vi "PlotTestData.vi"(0 "TestDataTable Ref":refnum<vi>, 1 "StopPlotDataEvn":refnum<user-event>, 2 "CleanDataEvn":refnum<user-event>, 3 "Powers Ref":refnum<vi>[](array[refnum]), 5 "TestDataCurve Ref":refnum<vi>, 7 "XAxis Ref":refnum<vi>, 9 "YAxes Ref":refnum<vi>[](array[refnum]), 11 "TestData2D":refnum<vi>, 12 "Setting":T1={"TorqueSensor"={"Interface"="", "Read Unit"=enum."Kg.cm", "Encoder"=0, "Torque Filter"=0, "Max Torque"=2.0, "Max Power"=50.0, "Max Speed"=50.0, "Scale Factor CW"=2.0, "Scale Factor CCW"=2.0, "Scale Factor Zero"=2.0}, "TorqueSensorL"={"Interface"="", "Read Unit"=enum."Kg.cm", "Encoder"=0, "Torque Filter"=0, "Max Torque"=2.0, "Max Power"=50.0, "Max Speed"=50.0, "Scale Factor CW"=2.0, "Scale Factor CCW"=2.0, "Scale Factor Zero"=2.0}, "Power Meter"={"Wiring"=0, "Interface"="", "1P Mode"=1, "1P CurrentLimit"=0.0, "3P Mode"=1, "3P CurrentLimit"=0.0}, "Thermocouple"={"Interface"="", "value range"="T/C T type -100 ~ 400 degree C", "Channel Count"=8, "Limit 0"=0.0, "Limit 1"=0.0, "Limit 2"=0.0, "Limit 3"=0.0, "Limit 4"=0.0, "Limit 5"=0.0, "Limit 6"=0.0, "Limit 7"=0.0}, "DC-1000"={"Interface"=enum."AD-1"}, "ServoMotor"={"Interface"=enum."AD-1"}, "MotorDriver"={"D_Interface"="", "L_Interface"=""}, "TestMode"=enum."電子中軸測試", "PowerSupply"={"Interface"="", "Current"=50.0, "Voltage"=50.0}, "DUTMotor"={"Active"=FALSE, "TPCANBaudrate"=enum."PCAN_BAUD_1M 0x0014"}} {"Thermocouple"."Limit 7" format="%.1f"; "Thermocouple"."Limit 6" format="%.1f"; "Thermocouple"."Limit 5" format="%.1f"; "Thermocouple"."Limit 4" format="%.1f"; "Thermocouple"."Limit 3" format="%.1f"; "Thermocouple"."Limit 2" format="%.1f"; "Thermocouple"."Limit 1" format="%.1f"; "Thermocouple"."Limit 0" format="%.1f"; "Thermocouple"."Channel Count" min=0 max=24; "Power Meter"."3P Mode" items=["RMS", "MEAN", "DC"]; "Power Meter"."1P Mode" items=["RMS", "MEAN", "DC"]; "Power Meter"."Wiring" items=["1P2W", "1P2W+3P3W3M"]; "TorqueSensorL"."Scale Factor Zero" format="%#.6f"; "TorqueSensorL"."Scale Factor CCW" format="%#.6f"; "TorqueSensorL"."Scale Factor CW" format="%#.6f"; "TorqueSensorL"."Torque Filter" items=["OFF", "10Hz", "25Hz", "50Hz", "3Hz", "2Hz", "1Hz"]; "TorqueSensorL"."Encoder" items=["60-ppr"=60, "600-ppr"=600, "6000-ppr"=6000, "8192-ppr"=8192, "20-ppr"=20, "30-ppr"=30, "1-ppr"=1, "2-ppr"=2, "6-ppr"=6]; "TorqueSensor"."Scale Factor Zero" format="%#.6f"; "TorqueSensor"."Scale Factor CCW" format="%#.6f"; "TorqueSensor"."Scale Factor CW" format="%#.6f"; "TorqueSensor"."Torque Filter" items=["OFF", "10Hz", "25Hz", "50Hz", "3Hz", "2Hz", "1Hz"]; "TorqueSensor"."Encoder" items=["60-ppr"=60, "600-ppr"=600, "6000-ppr"=6000, "8192-ppr"=8192, "20-ppr"=20, "30-ppr"=30, "1-ppr"=1, "2-ppr"=2, "6-ppr"=6]}, 13 "DataVisible Ref":refnum<vi>, 14 "Efficiency Ref":refnum<vi>) -> ()   [LabVIEW 2024]
uses:
  MFActor/SystemSettings.ctl
  ref/PCAN/CAN Communication.llb/TPCANBaudrate.ctl
  PlotTestDataStep.ctl
  <vilib>/Utility/error.llb/Trim Whitespace One-Sided.vi
  Global Variables.vi
panel:
  out "TestData1D 2":dbl[](array[numeric])
  out "DataNumber":u32
  out "StartTime":u32
  out "TestDataCurve":dbl[][](array[numeric])
  out "TestData1D":dbl[](array[numeric])
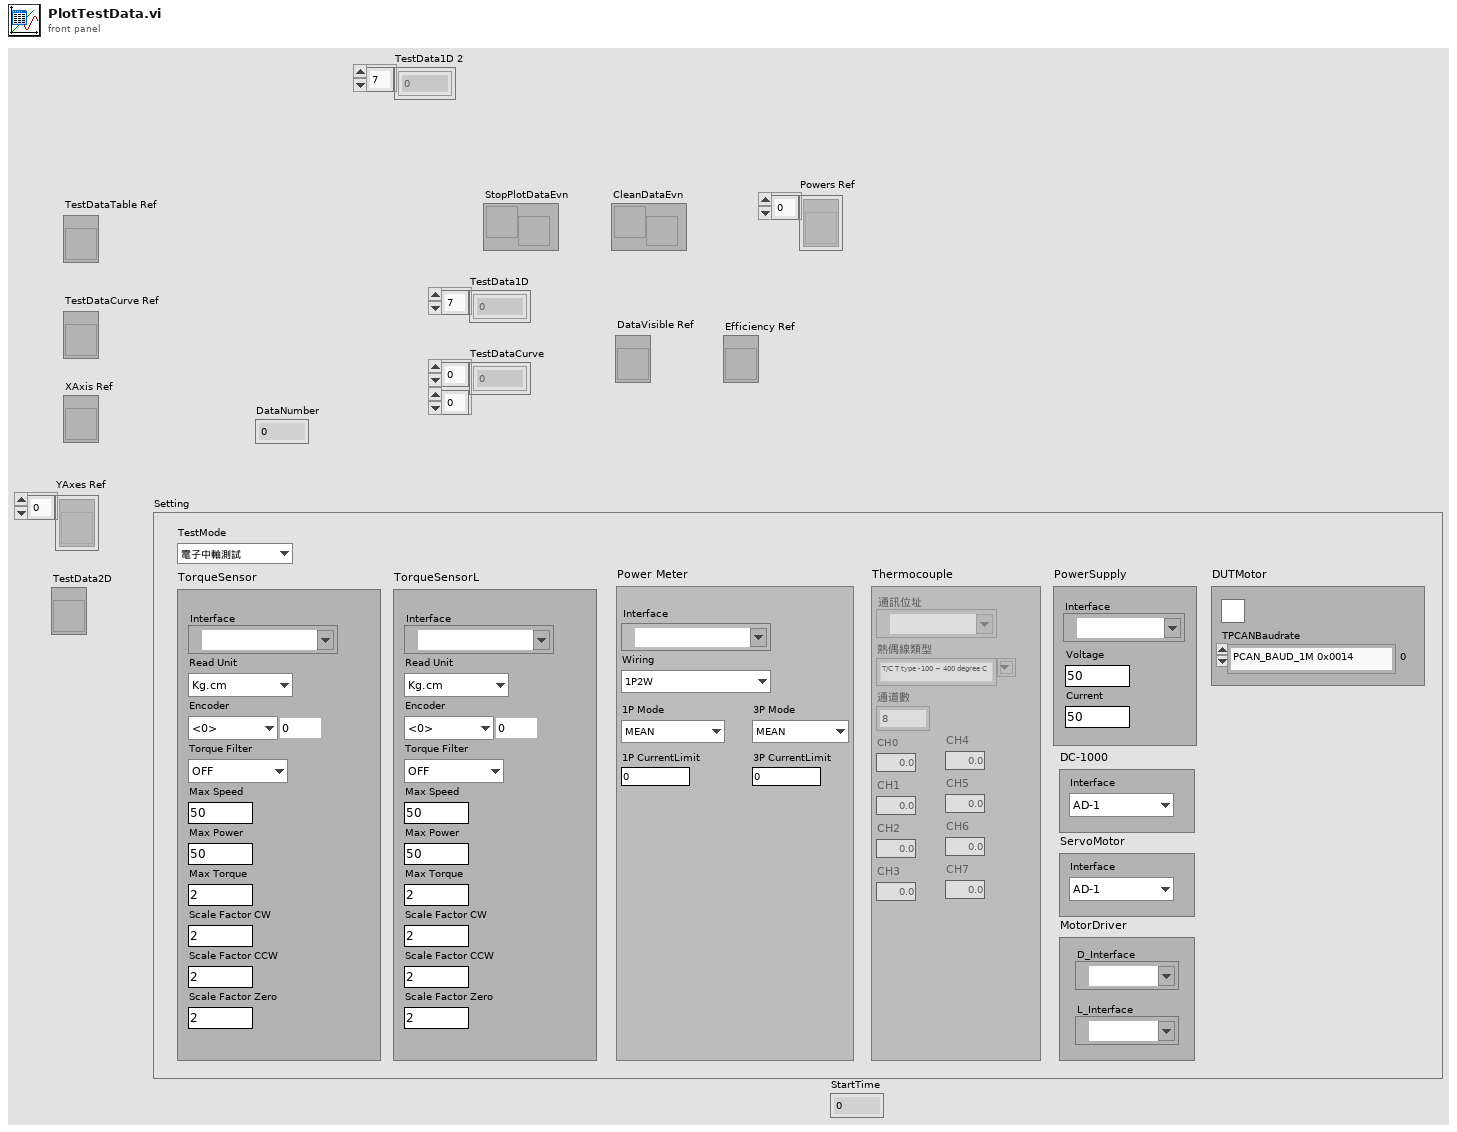
[diagram p1: front panel]
types:
  T1 = typedef "SystemSettings.ctl" = cluster{"TorqueSensor":cluster{"Interface":refnum<visa-resource-name>, "Read Unit":enum16{"oz.in", "oz.ft", "lb.in", "lb.ft", "g.cm", "Kg.cm", "mN.m", "cN.m", "N.m"}, "Encoder":u16, "Torque Filter":u16, "Max Torque":dbl, "Max Power":dbl, "Max Speed":dbl, "Scale Factor CW":dbl, "Scale Factor CCW":dbl, "Scale Factor Zero":dbl}, "TorqueSensorL":cluster{"Interface":refnum<visa-resource-name>, "Read Unit":enum16{"oz.in", "oz.ft", "lb.in", "lb.ft", "g.cm", "Kg.cm", "mN.m", "cN.m", "N.m"}, "Encoder":u16, "Torque Filter":u16, "Max Torque":dbl, "Max Power":dbl, "Max Speed":dbl, "Scale Factor CW":dbl, "Scale Factor CCW":dbl, "Scale Factor Zero":dbl}, "Power Meter":cluster{"Wiring":u16, "Interface":refnum<visa-resource-name>, "1P Mode":u16, "1P CurrentLimit":dbl, "3P Mode":u16, "3P CurrentLimit":dbl}, "Thermocouple":cluster{"Interface":refnum<visa-resource-name>, "value range":string, "Channel Count":i32, "Limit 0":dbl, "Limit 1":dbl, "Limit 2":dbl, "Limit 3":dbl, "Limit 4":dbl, "Limit 5":dbl, "Limit 6":dbl, "Limit 7":dbl}, "DC-1000":cluster{"Interface":enum16{"AD-0", "AD-1"}}, "ServoMotor":cluster{"Interface":enum16{"AD-0", "AD-1"}}, "MotorDriver":cluster{"D_Interface":refnum<visa-resource-name>, "L_Interface":refnum<visa-resource-name>}, "TestMode":enum16{"電子中軸測試", "中置電機測試"}, "PowerSupply":cluster{"Interface":refnum<visa-resource-name>, "Current":dbl, "Voltage":dbl}, "DUTMotor":cluster{"Active":bool, "TPCANBaudrate":T2}}
  T2 = typedef "TPCANBaudrate.ctl" = enum16{"PCAN_BAUD_1M 0x0014", "PCAN_BAUD_800K 0x0016", "PCAN_BAUD_500K 0x001C", "PCAN_BAUD_250K 0x011C", "PCAN_BAUD_125K 0x031C", "PCAN_BAUD_100K 0x432F", "PCAN_BAUD_95K 0xC34E", "PCAN_BAUD_83K 0x852B", "PCAN_BAUD_50K 0x472F", "PCAN_BAUD_47K 0x1414", "PCAN_BAUD_33K 0x8B2F", "PCAN_BAUD_20K 0x532F", "PCAN_BAUD_10K 0x672F", "PCAN_BAUD_5K 0x7F7F", "User Baudrate"}
  T3 = cluster{"GraphTestData":dbl[], "GraphTestData 2":dbl[]}[]
  T4 = typedef "PlotTestDataStep.ctl" = enum16{"None", "CheckTestData", "CalculateEffi", "Plot", "DataVisible", "UpdateGraph", "Clean", "End"}
  T5 = cluster{"SR":dbl, "EffiDriver":dbl, "EffiMotor":dbl, "EffiTotal":dbl}
  T6 = cluster{"TestDataCurve":dbl[], "TestDataCurve":dbl[]}
  T7 = cluster{"TestDataCurve":dbl[], "TestDataCurve":dbl[]}[]
  T8 = typedef "LVRowAndColumnUnsignedTypeDef.ctl" = cluster{"Row":u32, "Column":u32}
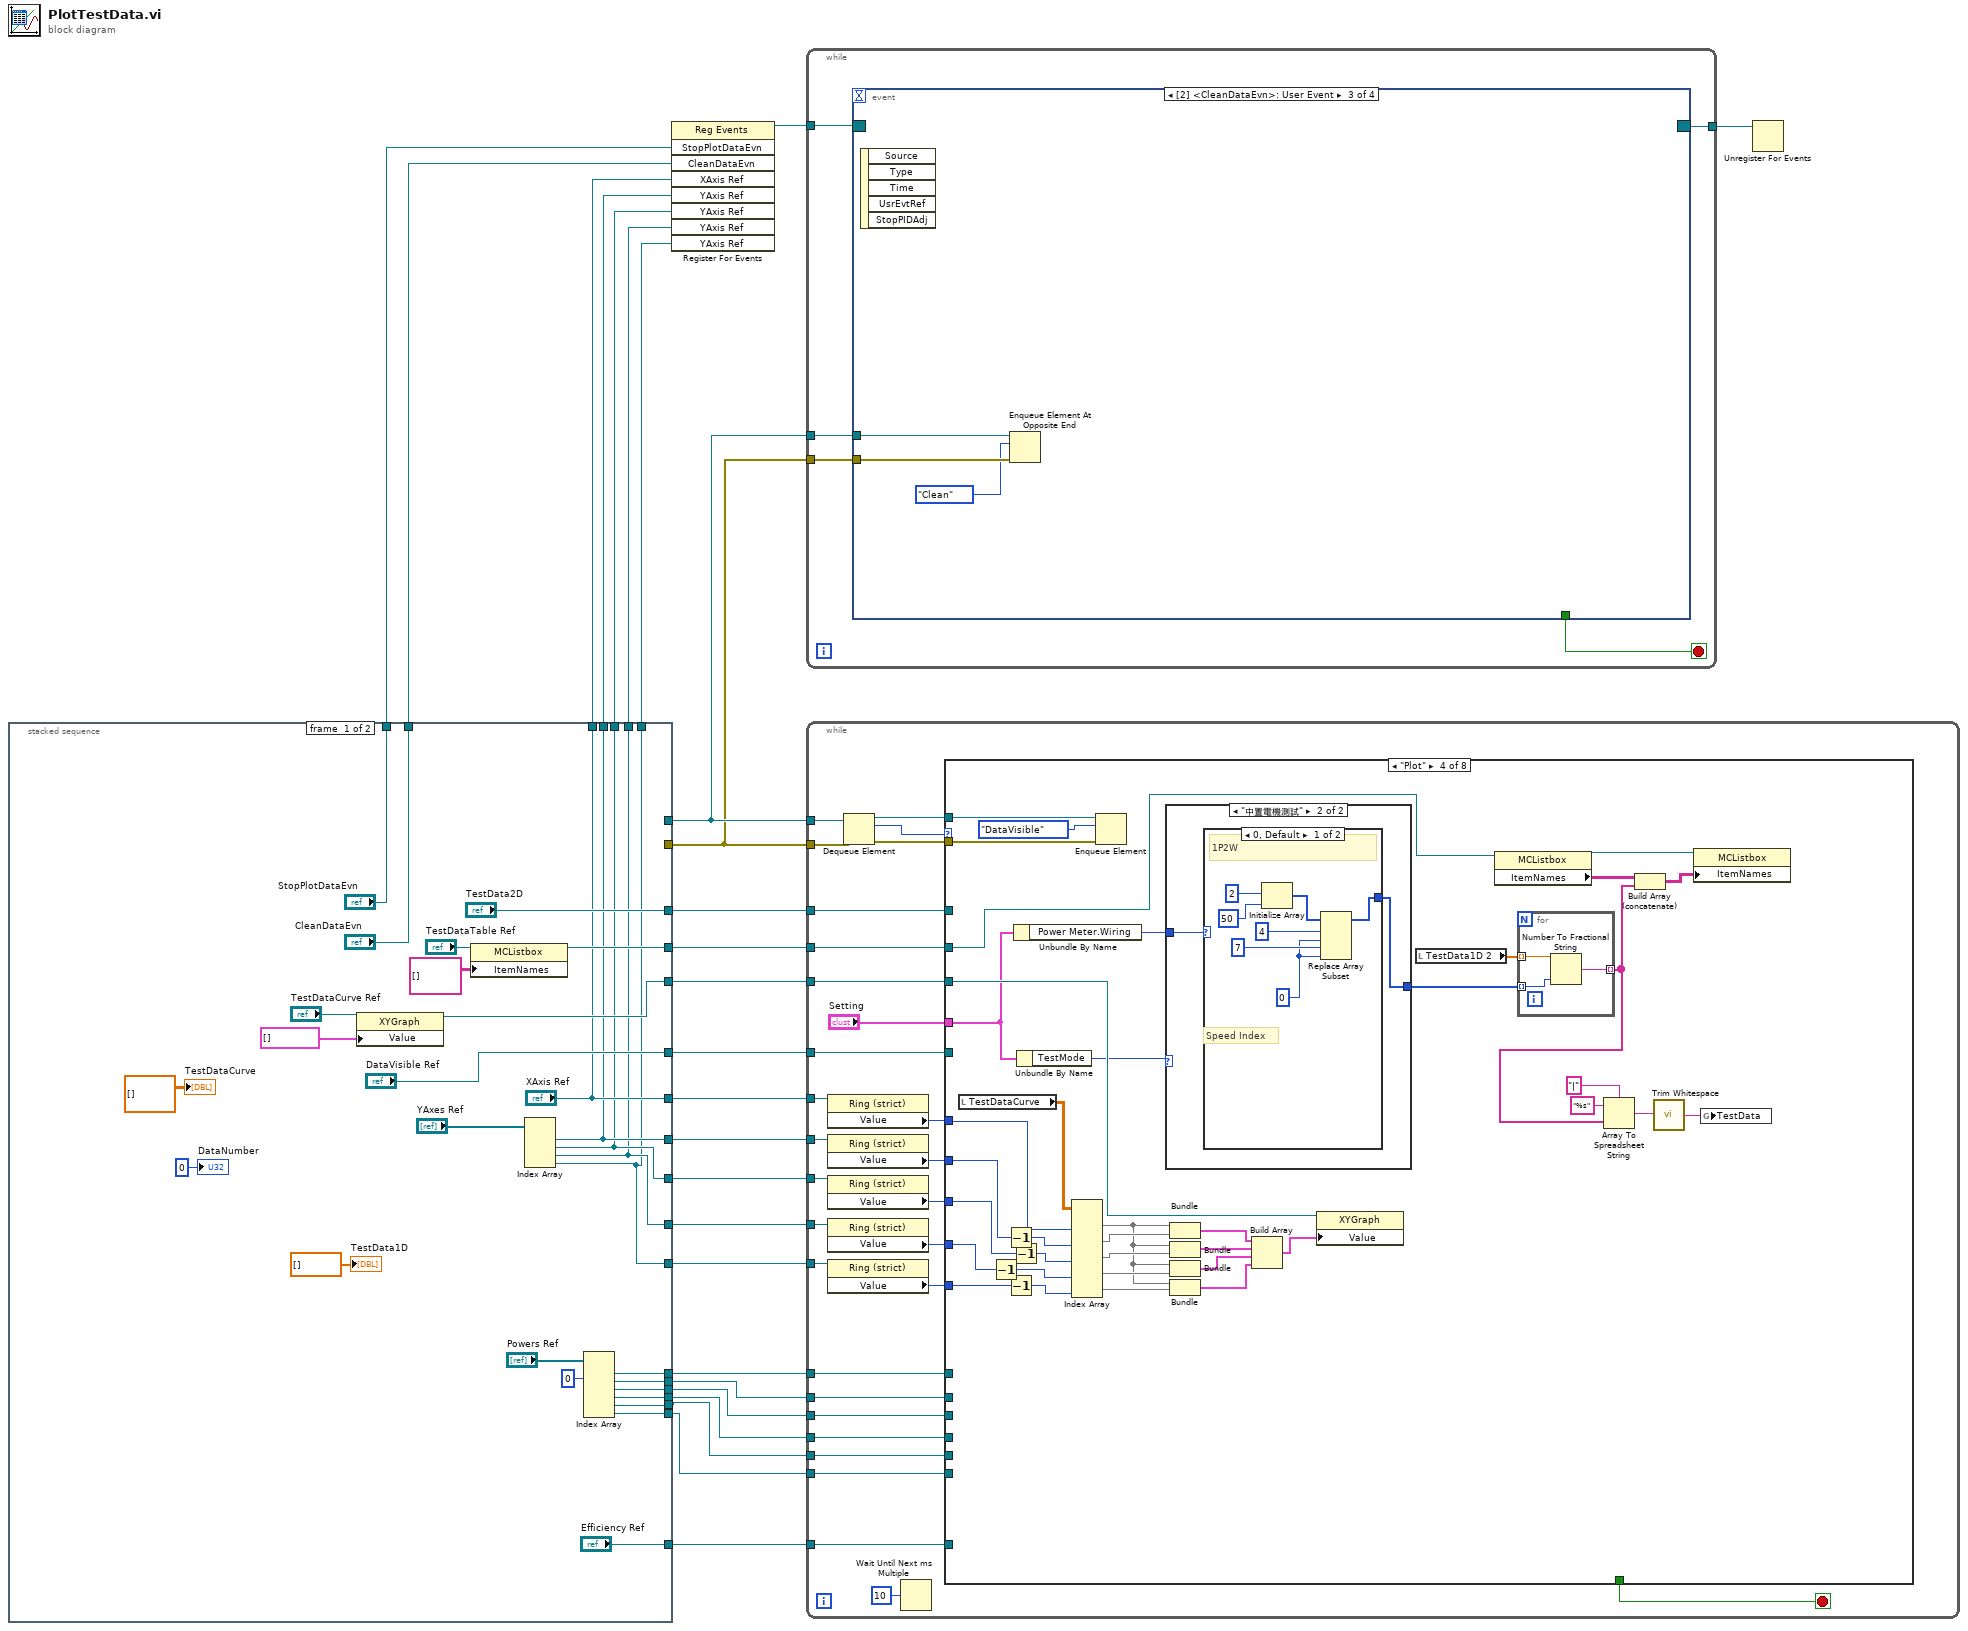
[diagram p0: block diagram]
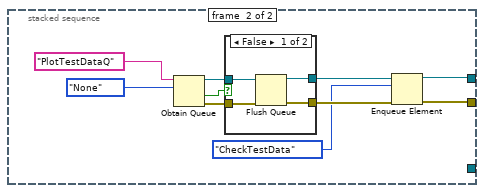
[diagram p2: hidden frame]
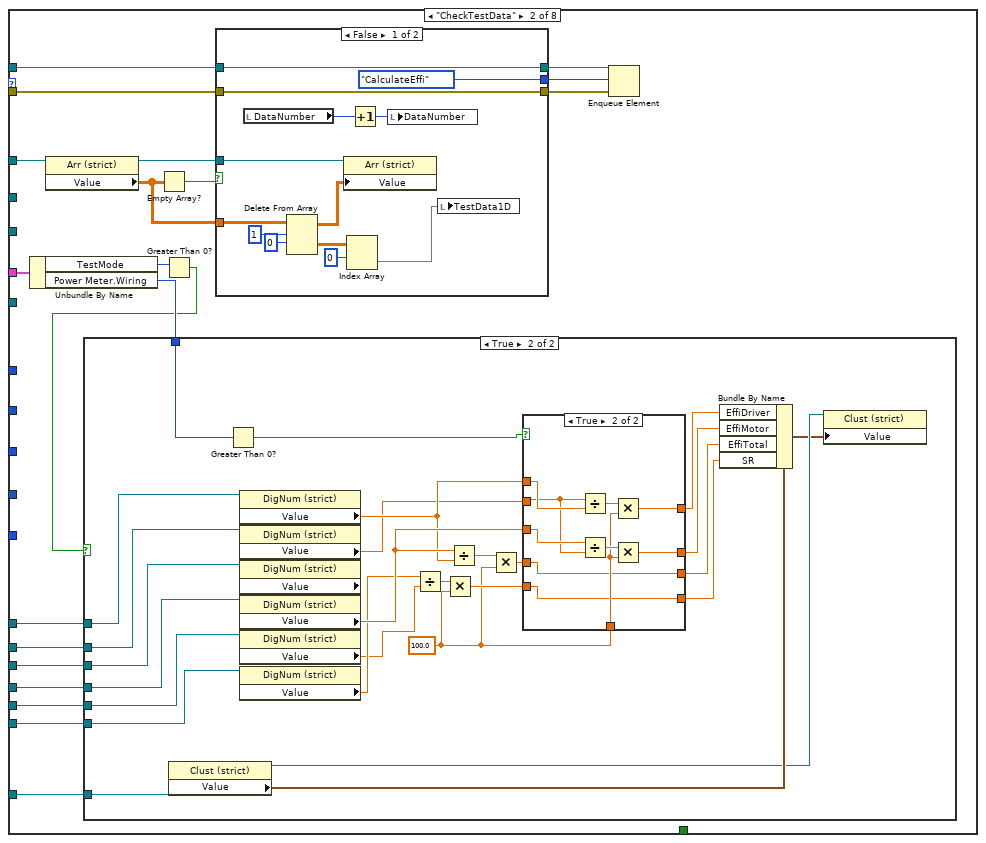
[diagram p5: hidden frame]
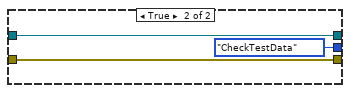
[diagram p8: hidden frame]
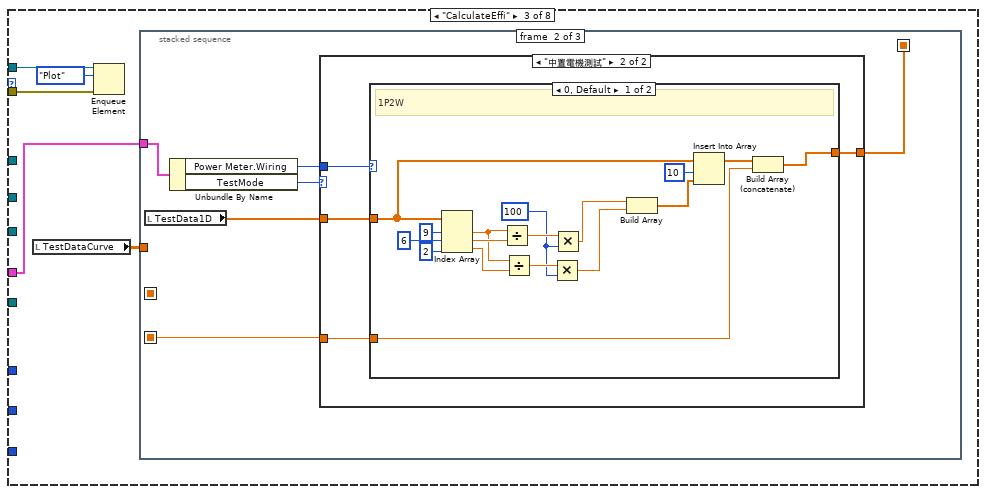
[diagram p9: hidden frame]
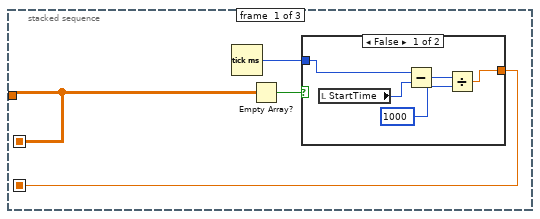
[diagram p10: hidden frame]
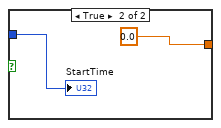
[diagram p11: hidden frame]
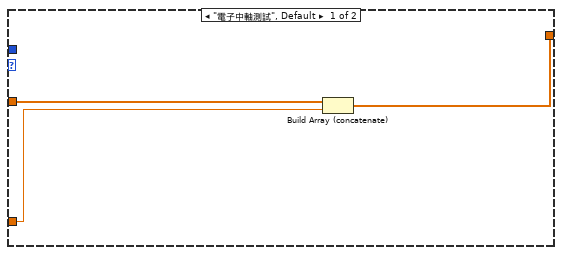
[diagram p12: hidden frame]
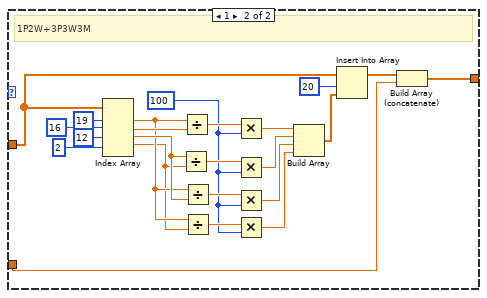
[diagram p13: hidden frame]
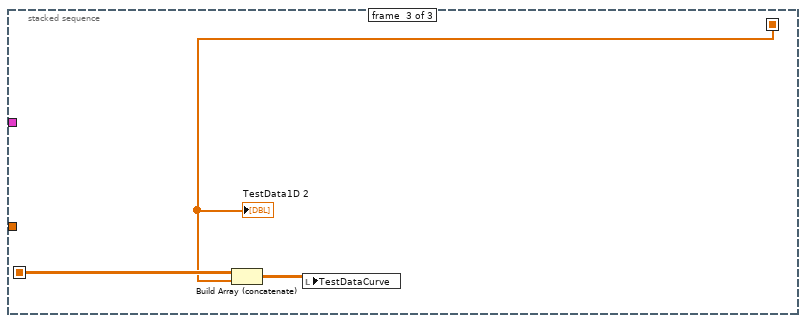
[diagram p14: hidden frame]
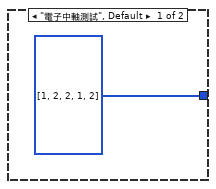
[diagram p15: hidden frame]
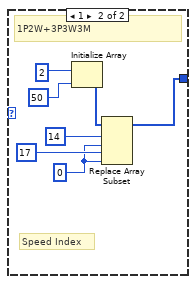
[diagram p16: hidden frame]
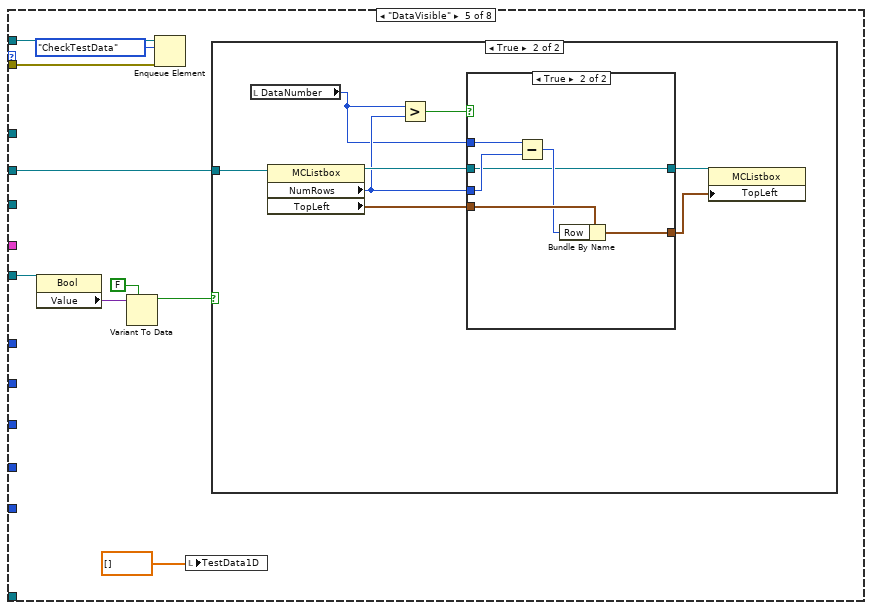
[diagram p17: hidden frame]
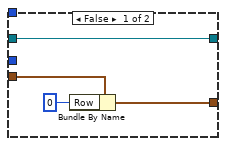
[diagram p19: hidden frame]
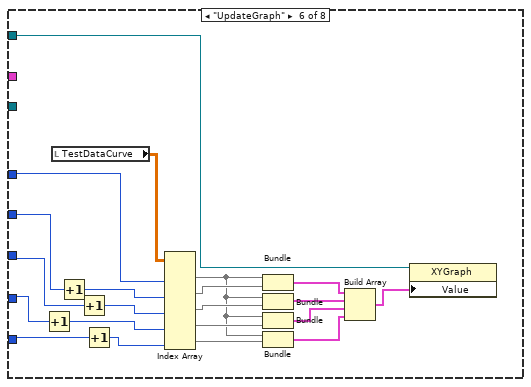
[diagram p20: hidden frame]
diagram:
  n1 = stacked-sequence {
    tunnel: ["StopPlotDataEvn" _] -> w27
    tunnel: ["CleanDataEvn" _] -> w26
    tunnel: [_ w58] -> w24
    tunnel: [_ w57] -> w23
    tunnel: ["TestData2D" _] -> w22
    tunnel: [w50 _] -> w21
    tunnel: [w47 _] -> w20
    tunnel: ["XAxis Ref" _] -> w19
    tunnel: [w41 _] -> w18
    tunnel: [w40 _] -> w17
    tunnel: [w39 _] -> w16
    tunnel: [w38 _] -> w15
    tunnel: ["DataVisible Ref" _] -> w13
    tunnel: ["XAxis Ref" _] -> w12
    tunnel: [w41 _] -> w11
    tunnel: [w40 _] -> w10
    tunnel: [w39 _] -> w9
    tunnel: [w38 _] -> w8
    tunnel: [w35 _] -> w7
    tunnel: [w34 _] -> w6
    tunnel: [w33 _] -> w5
    tunnel: [w32 _] -> w4
    tunnel: ["Efficiency Ref" _] -> w3
    tunnel: [w29 _] -> w2
    tunnel: [w28 _] -> w1
    frame #0 {
      n2 = property class="XYGraph"(reference="TestDataCurve Ref", "Value"=T3 []) -> (reference out=w47:refnum<vi>)  [unwired: 1 in, 1 out]
      n3 = property class="MCListbox"(reference="TestDataTable Ref", "ItemNames"=string[][] [] ("Item Names")) -> (reference out=w50:refnum<vi>)  [unwired: 1 in, 1 out]
      n4 = Index Array(array="YAxes Ref") -> (element #1=w41:refnum<vi>, element #2=w40:refnum<vi>, element #3=w39:refnum<vi>, element #4=w38:refnum<vi>)  [unwired: 4 in]
      n5 = Index Array(array="Powers Ref", index #1=0 ("index")) -> (element #1=w35:refnum<vi>, element #2=w34:refnum<vi>, element #3=w33:refnum<vi>, element #4=w32:refnum<vi>, element #5=w29:refnum<vi>, element #6=w28:refnum<vi>)  [unwired: 5 in]
      "TestDataCurve" <- dbl[][] [] ("TestData2D")
      "DataNumber" <- u32 0 ("DataNumber")
      "TestData1D" <- dbl[] [] ("TestData1D")
    }
    frame #1 {
      n6 = Obtain Queue(name (unnamed)="PlotTestDataQ", element data type=PlotTestDataStep."None" ("PlotTestDataStep")) -> (queue out=w62:refnum<queue>, created new?=w63:bool, error out=w61:errorcluster)  [unwired: 3 in]
      n7 = case shown="False" w63 {
        tunnel: w62 -> [w69 w71]
        tunnel: w61 -> [w68 w70]
        tunnel: [w67 w71] -> w60
        tunnel: [w66 w70] -> w59
        frame False {
          n8 = Flush Queue(queue=w69, error in (no error)=w68) -> (queue out=w67:refnum<queue>, error out=w66:errorcluster)  [unwired: 1 out]
        }
        frame True {
        }
      }
      n9 = Enqueue Element(queue=w60, element=PlotTestDataStep."CheckTestData", error in (no error)=w59) -> (queue out=w58:refnum<queue>, error out=w57:errorcluster)  [unwired: 1 in, 1 out]
    }
  }
  n10 = register-events(w27, w26, w12, w11, w10, w9, w8) -> (reference out=w25:refnum<event-registration>)  [unwired: 2 in, 1 out]
  n11 = while {
    tunnel: w25 -> [w76]
    tunnel: w24 -> [w75]
    tunnel: w23 -> [w74]
    tunnel: [w72] -> w14
    stop <- w73 stop-if-true
    n12 = event shown="[2] <CleanDataEvn>: User Event" {
      selector: w76 -> [_ _ _ _]
      dyn-events: [_ _ _ _] -> w72
      timeout: _ -> [_ _ _ _]
      tunnel: w75 -> [_ w82 w85 w88]
      tunnel: w74 -> [_ w81 w84 w87]
      tunnel: [_ TRUE _ _] -> w73
      event Timeout {
        n13 = event-data() -> ()  [unwired: 1 in, 3 out]
      }
      event User Event {
        n14 = event-data() -> ()  [unwired: 1 in, 5 out]
        n15 = Flush Queue(queue=w82, error in (no error)=w81) -> (queue out=w80:refnum<queue>, error out=w79:errorcluster)  [unwired: 1 out]
        n16 = Enqueue Element At Opposite End(queue=w80, element=PlotTestDataStep."End", error in (no error)=w79) -> ()  [unwired: 1 in, 3 out]
      }
      event User Event {
        n17 = event-data() -> ()  [unwired: 1 in, 5 out]
        n18 = Enqueue Element At Opposite End(queue=w85, element=PlotTestDataStep."Clean", error in (no error)=w84) -> ()  [unwired: 1 in, 3 out]
      }
      event Value Change {
        n19 = event-data() -> ()  [unwired: 1 in, 6 out]
        n20 = Enqueue Element(queue=w88, element=PlotTestDataStep."UpdateGraph", error in (no error)=w87) -> ()  [unwired: 1 in, 3 out]
      }
    }
  }
  n21 = while {
    tunnel: w24 -> [w117]
    tunnel: w23 -> [w116]
    tunnel: w22 -> [w110]
    tunnel: w21 -> [w108]
    tunnel: w20 -> [w97]
    tunnel: w19 -> [w99]
    tunnel: w18 -> [w107]
    tunnel: w17 -> [w106]
    tunnel: w16 -> [w105]
    tunnel: w15 -> [w104]
    tunnel: w13 -> [w96]
    tunnel: w7 -> [w94]
    tunnel: w6 -> [w93]
    tunnel: w5 -> [w92]
    tunnel: w4 -> [w91]
    tunnel: w3 -> [w95]
    tunnel: w2 -> [w90]
    tunnel: w1 -> [w89]
    stop <- w111 stop-if-true
    n22 = property class="Ring (strict)"(reference=w99) -> ("Value"=w98:u16)  [unwired: 1 in, 2 out]
    n23 = property class="Ring (strict)"(reference=w107) -> ("Value"=w103:u16)  [unwired: 1 in, 2 out]
    n24 = property class="Ring (strict)"(reference=w106) -> ("Value"=w102:u16)  [unwired: 1 in, 2 out]
    n25 = property class="Ring (strict)"(reference=w105) -> ("Value"=w101:u16)  [unwired: 1 in, 2 out]
    n26 = property class="Ring (strict)"(reference=w104) -> ("Value"=w100:u16)  [unwired: 1 in, 2 out]
    n27 = Dequeue Element(queue=w117, error in (no error)=w116) -> (queue out=w115:refnum<queue>, element=w113:T4, error out=w114:errorcluster)  [unwired: 1 in, 1 out]
    n28 = Wait Until Next ms Multiple(millisecond multiple=u32 10) -> ()  [unwired: 1 out]
    n29 = case shown="\"Plot\"" w113 {
      tunnel: w115 -> [_ w133 w196 w279 w325 _ _ w383]
      tunnel: w114 -> [_ w132 w195 w278 w324 _ _ w382]
      tunnel: [_ _ _ _ _ _ _ TRUE] -> w111
      tunnel: w110 -> [_ w137 _ _ _ _ _ _]
      tunnel: "Setting" -> [_ w124 w193 w276 _ _ _ _]
      tunnel: w108 -> [_ _ _ w299 w326 _ w376 _]
      tunnel: w103 -> [_ _ _ w294 _ w356 _ _]
      tunnel: w102 -> [_ _ _ w293 _ w357 _ _]
      tunnel: w101 -> [_ _ _ w292 _ w358 _ _]
      tunnel: w100 -> [_ _ _ w291 _ w359 _ _]
      tunnel: w98 -> [_ _ _ w265 _ w353 _ _]
      tunnel: w97 -> [_ _ _ w281 _ w354 w374 _]
      tunnel: w96 -> [_ _ _ _ w330 _ _ _]
      tunnel: w95 -> [_ w121 _ _ _ _ _ _]
      tunnel: w94 -> [_ w128 _ _ _ _ _ _]
      tunnel: w93 -> [_ w127 _ _ _ _ _ _]
      tunnel: w92 -> [_ w126 _ _ _ _ _ _]
      tunnel: w91 -> [_ w125 _ _ _ _ _ _]
      tunnel: w90 -> [_ w119 _ _ _ _ _ _]
      tunnel: w89 -> [_ w118 _ _ _ _ _ _]
      frame "None", Default {
      }
      frame "CheckTestData" {
        n30 = Unbundle By Name(w124) -> ("TestMode"=w123:enum16{"電子中軸測試", "中置電機測試"}, "Power Meter.Wiring"=w122:u16)
        n31 = property class="Arr (strict)"(reference=w137) -> (reference out=w134:refnum<vi>, "Value"=w135:dbl[][])  [unwired: 1 in, 1 out]
        n32 = Empty Array?(array=w135) -> (empty?=w136:bool)
        n33 = Greater Than 0?(x=w123) -> (x > 0?=w120:bool)
        n34 = case shown="True" w120 {
          tunnel: w128 -> [_ w163]
          tunnel: w127 -> [_ w162]
          tunnel: w126 -> [_ w161]
          tunnel: w125 -> [_ w160]
          tunnel: w122 -> [_ w157]
          tunnel: w121 -> [_ w149]
          tunnel: w119 -> [_ w141]
          tunnel: w118 -> [_ w140]
          frame False {
          }
          frame True {
            w151 = 100.0 ("y")
            n35 = property class="Clust (strict)"(reference=w149) -> (reference out=w143:refnum<vi>, "Value"=w148:T5)  [unwired: 1 in, 1 out]
            n36 = Greater Than 0?(x=w157) -> (x > 0?=w156:bool)
            n37 = property class="DigNum (strict)"(reference=w163) -> ("Value"=w152:dbl)  [unwired: 1 in, 2 out]
            n38 = property class="DigNum (strict)"(reference=w162) -> ("Value"=w150:dbl)  [unwired: 1 in, 2 out]
            n39 = property class="DigNum (strict)" props=["Value"](reference=w161) -> ()  [unwired: 1 in, 3 out]
            n40 = property class="DigNum (strict)"(reference=w160) -> ("Value"=w153:dbl)  [unwired: 1 in, 2 out]
            n41 = property class="DigNum (strict)"(reference=w141) -> ("Value"=w138:dbl)  [unwired: 1 in, 2 out]
            n42 = property class="DigNum (strict)"(reference=w140) -> ("Value"=w139:dbl)  [unwired: 1 in, 2 out]
            n43 = Divide(x=w139, y=w138) -> (x/y=w159:dbl)
            n44 = Multiply(x=w159, y=w151) -> (x*y=w154:dbl)
            n45 = Divide(x=w153, y=w152) -> (x/y=w158:dbl)
            n46 = Multiply(x=w158, y=w151) -> (x*y=w155:dbl)
            n47 = case shown="True" w156 {
              tunnel: w155 -> [w165 w167]
              tunnel: w154 -> [w164 w166]
              tunnel: w153 -> [_ w172]
              tunnel: w152 -> [_ w174]
              tunnel: w151 -> [_ w170]
              tunnel: w150 -> [_ w171]
              tunnel: [_ w169] -> w147
              tunnel: [_ w168] -> w146
              tunnel: [w165 w167] -> w145
              tunnel: [w164 w166] -> w144
              frame False {
              }
              frame True {
                n48 = Divide(x=w171, y=w174) -> (x/y=w175:dbl)
                n49 = Divide(x=w172, y=w171) -> (x/y=w173:dbl)
                n50 = Multiply(x=w175, y=w170) -> (x*y=w169:dbl)
                n51 = Multiply(x=w173, y=w170) -> (x*y=w168:dbl)
              }
            }
            n52 = Bundle By Name(cluster=w148, "EffiDriver"=w147, "EffiMotor"=w146, "EffiTotal"=w145, "SR"=w144) -> (w142:T5)
            n53 = property class="Clust (strict)"(reference=w143, "Value"=w142) -> ()  [unwired: 1 in, 2 out]
          }
        }
        n54 = case shown="False" w136 {
          tunnel: w135 -> [w188 _]
          tunnel: w134 -> [w185 _]
          tunnel: w133 -> [w181 w191]
          tunnel: w132 -> [w180 w190]
          tunnel: [w181 w191] -> w131
          tunnel: [w180 w190] -> w130
          tunnel: [PlotTestDataStep."CalculateEffi" ("element") PlotTestDataStep."CheckTestData" ("element")] -> w129
          frame False {
            n55 = local read "DataNumber"() -> (w178:u32)
            n56 = Delete From Array(array=w188, length=1, index (row)=0) -> (deleted portion=w183:dbl[][], array with subset deleted=w184:dbl[][])  [unwired: 1 in]
            n57 = property class="Arr (strict)"(reference=w185, "Value"=w184) -> ()  [unwired: 1 in, 2 out]
            n58 = Index Array(array=w183, index (row)=0) -> (element=w176:dbl[])  [unwired: 1 in]
            n59 = Increment(x=w178) -> (x+1=w177:u32)
            n60 = local write "DataNumber"(w177) -> ()
            n61 = local write "TestData1D"(w176) -> ()
          }
          frame True {
          }
        }
        n62 = Enqueue Element(queue=w131, element=w129, error in (no error)=w130) -> ()  [unwired: 1 in, 3 out]
      }
      frame "CalculateEffi" {
        n63 = local read "TestDataCurve"() -> (w192:dbl[][])
        n64 = Enqueue Element(queue=w196, element=PlotTestDataStep."Plot", error in (no error)=w195) -> ()  [unwired: 1 in, 3 out]
        n65 = stacked-sequence {
          seq-local: [w198 _ _] -> [_ w209 _]
          seq-local: [w197 _ _] -> [_ _ w263]
          seq-local: [_ w208 _] -> [_ _ w261]
          tunnel: w193 -> [_ w212 _]
          tunnel: w192 -> [w197 _ _]
          frame #0 {
            n66 = Tick Count (ms)() -> (millisecond timer value=w200:u32)
            n67 = Empty Array?(array=w197) -> (empty?=w199:bool)
            n68 = case shown="False" w199 {
              tunnel: w200 -> [w205 w207]
              tunnel: [w201 0.0] -> w198
              frame False {
                n69 = local read "StartTime"() -> (w204:u32)
                n70 = Subtract(x=w205, y=w204) -> (x-y=w203:u32)
                n71 = Divide(x=w203, y=u32 1000) -> (x/y=w201:dbl)
              }
              frame True {
                "StartTime" <- w207
              }
            }
          }
          frame #1 {
            n72 = local read "TestData1D"() -> (w213:dbl[])
            n73 = Unbundle By Name(w212) -> ("Power Meter.Wiring"=w210:u16, "TestMode"=w211:enum16{"電子中軸測試", "中置電機測試"})
            n74 = case shown="\"中置電機測試\"" w211 {
              tunnel: w213 -> [w216 w220]
              tunnel: w209 -> [w215 w217]
              tunnel: [w214 w219] -> w208
              tunnel: w210 -> [_ w218]
              frame "電子中軸測試", Default {
                n75 = Build Array (concatenate)(w216, w215) -> (w214:dbl[])
              }
              frame "中置電機測試" {
                n76 = case shown="0, Default" w218 {
                  tunnel: w220 -> [w226 w243]
                  tunnel: w217 -> [w222 w239]
                  tunnel: [w221 w238] -> w219
                  frame 0, Default {
                    w229 = 100
                    # "1P2W"
                    n77 = Index Array(array=w226, index #1=9 ("index"), index #2=6 ("index"), index #3=2 ("index")) -> (element #1=w233:dbl, element #2=w235:dbl, element #3=w232:dbl)
                    n78 = Divide(x=w233, y=w235) -> (x/y=w231:dbl)
                    n79 = Divide(x=w233, y=w232) -> (x/y=w230:dbl)
                    n80 = Multiply(x=w230, y=w229) -> (x*y=w227:dbl)
                    n81 = Multiply(x=w231, y=w229) -> (x*y=w228:dbl)
                    n82 = Build Array(w228, w227) -> (w224:dbl[])
                    n83 = Insert Into Array(array=w226, index=10, new element=w224) -> (w223:dbl[])
                    n84 = Build Array (concatenate)(w223, w222) -> (w221:dbl[])
                  }
                  frame 1 {
                    w248 = 100
                    # "1P2W+3P3W3M"
                    n85 = Index Array(array=w243, index #1=19 ("index"), index #2=16 ("index"), index #3=12 ("index"), index #4=2 ("index")) -> (element #1=w254:dbl, element #2=w258:dbl, element #3=w255:dbl, element #4=w253:dbl)  [unwired: 1 in, 1 out]
                    n86 = Divide(x=w255, y=w253) -> (x/y=w251:dbl)
                    n87 = Divide(x=w254, y=w258) -> (x/y=w252:dbl)
                    n88 = Divide(x=w254, y=w255) -> (x/y=w250:dbl)
                    n89 = Divide(x=w254, y=w253) -> (x/y=w249:dbl)
                    n90 = Multiply(x=w252, y=w248) -> (x*y=w247:dbl)
                    n91 = Multiply(x=w251, y=w248) -> (x*y=w246:dbl)
                    n92 = Multiply(x=w250, y=w248) -> (x*y=w245:dbl)
                    n93 = Multiply(x=w249, y=w248) -> (x*y=w244:dbl)
                    n94 = Build Array(w247, w246, w245, w244) -> (w241:dbl[])
                    n95 = Insert Into Array(array=w243, index=20, new element=w241) -> (w240:dbl[])
                    n96 = Build Array (concatenate)(w240, w239) -> (w238:dbl[])
                  }
                }
              }
            }
          }
          frame #2 {
            n97 = Build Array (concatenate)(w263, w261) -> (w262:dbl[][])
            n98 = local write "TestDataCurve"(w262) -> ()
            "TestData1D 2" <- w261
          }
        }
      }
      frame "Plot" {
        n99 = local read "TestDataCurve"() -> (w295:dbl[][])
        n100 = Decrement(x=w292) -> (x-1=w268:u16)
        n101 = Decrement(x=w294) -> (x-1=w266:u16)
        n102 = Decrement(x=w291) -> (x-1=w269:u16)
        n103 = Decrement(x=w293) -> (x-1=w267:u16)
        n104 = Unbundle By Name(w276) -> ("Power Meter.Wiring"=w301:u16)
        n105 = Unbundle By Name(w276) -> ("TestMode"=w275:enum16{"電子中軸測試", "中置電機測試"})
        n106 = Index Array(array=w295, index (col) #1=w265, index (col) #2=w266, index (col) #3=w267, index (col) #4=w268, index (col) #5=w269) -> (element #1=w286:dbl[], element #2=w287:dbl[], element #3=w288:dbl[], element #4=w289:dbl[], element #5=w290:dbl[])  [unwired: 5 in]
        n107 = Enqueue Element(queue=w279, element=PlotTestDataStep."DataVisible", error in (no error)=w278) -> ()  [unwired: 1 in, 3 out]
        n108 = case shown="\"中置電機測試\"" w275 {
          tunnel: w301 -> [_ w307]
          tunnel: [i32[] [1, 2, 2, 1, 2] w306] -> w300
          frame "電子中軸測試", Default {
          }
          frame "中置電機測試" {
            n109 = case shown="0, Default" w307 {
              tunnel: [w310 w315] -> w306
              frame 0, Default {
                w308 = 0 ("new element/subarray")
                # "Speed Index"
                # "1P2W"
                n110 = Initialize Array(2, 50 ("dimension size")) -> (w312:i32[])
                n111 = Replace Array Subset(array=w312, new element #1=w308, index #1=4 ("index"), new element #2=w308, index #2=7 ("index")) -> (w310:i32[])
              }
              frame 1 {
                w316 = 0 ("new element/subarray")
                # "Speed Index"
                # "1P2W+3P3W3M"
                n112 = Initialize Array(2, 50 ("dimension size")) -> (w319:i32[])
                n113 = Replace Array Subset(array=w319, new element #1=w316, index #1=14 ("index"), new element #2=w316, index #2=17 ("index")) -> (w315:i32[])
              }
            }
          }
        }
        n114 = Bundle("TestDataCurve"=w286, "TestDataCurve"=w287) -> (w285:T6)  [unwired: 1 in]
        n115 = Bundle("TestDataCurve"=w286, "TestDataCurve"=w288) -> (w284:T6)  [unwired: 1 in]
        n116 = Bundle("TestDataCurve"=w286, "TestDataCurve"=w289) -> (w283:T6)  [unwired: 1 in]
        n117 = Bundle("TestDataCurve"=w286, "TestDataCurve"=w290) -> (w282:T6)  [unwired: 1 in]
        n118 = Build Array(w285, w284, w283, w282) -> (w280:T7)
        n119 = property class="XYGraph"(reference=w281, "Value"=w280) -> ()  [unwired: 1 in, 2 out]
        n120 = local read "TestData1D 2"() -> (w264:dbl[])
        n121 = property class="MCListbox"(reference=w299) -> (reference out=w297:refnum<vi>, "ItemNames"=w298:string[][])  [unwired: 1 in, 1 out]
        n122 = for {
          tunnel: w300 -> [w303] mode=indexing
          tunnel: w264 -> [w304] mode=indexing
          tunnel: [w302] -> w270 mode=indexing
          n123 = Number To Fractional String(number=w304, precision (6)=w303) -> (F-format string=w302:string)  [unwired: 2 in]
        }
        n124 = Array To Spreadsheet String(delimiter (Tab)="|", array=w270, 3:"%s" ("format string")) -> (spreadsheet string=w271:string)
        n125 = Build Array (concatenate)(w298, w270) -> (w296:string[][])
        n126 = call <vilib>:"Trim Whitespace.vi"("string"=w271) -> ("trimmed string"=w274:string)  [unwired: 1 in]
        n127 = property class="MCListbox"(reference=w297, "ItemNames"=w296) -> ()  [unwired: 1 in, 2 out]
        n128 = global write "Global Variables.vi" "TestData"(w274) -> ()
      }
      frame "DataVisible" {
        n129 = property class="Bool"(reference=w330) -> ("Value"=w329:variant)  [unwired: 1 in, 2 out]
        n130 = Variant To Data(type=FALSE, Variant=w329) -> (data=w327:bool)  [unwired: 1 in, 1 out]
        n131 = Enqueue Element(queue=w325, element=PlotTestDataStep."CheckTestData", error in (no error)=w324) -> ()  [unwired: 1 in, 3 out]
        n132 = local write "TestData1D"(dbl[] [] ("TestDataCurve")) -> ()
        n133 = case shown="True" w327 {
          tunnel: w326 -> [_ w338]
          frame False {
          }
          frame True {
            n134 = local read "DataNumber"() -> (w331:u32)
            n135 = property class="MCListbox"(reference=w338) -> (reference out=w335:refnum<vi>, "NumRows"=w332:u32, "TopLeft"=w336:T8)  [unwired: 1 in, 1 out]
            n136 = Greater?(x=w331, y=w332) -> (0:w337:bool)
            n137 = case shown="True" w337 {
              tunnel: w336 -> [w341 w346]
              tunnel: [w340 w344] -> w333
              tunnel: w335 -> [w339 w343]
              tunnel: [w339 w343] -> w334
              tunnel: w332 -> [_ w347]
              tunnel: w331 -> [_ w348]
              frame False {
                n138 = Bundle By Name(cluster=w341, "Row"=u32 0) -> (w340:T8)
              }
              frame True {
                n139 = Subtract(x=w348, y=w347) -> (x-y=w345:u32)
                n140 = Bundle By Name(cluster=w346, "Row"=w345) -> (w344:T8)
              }
            }
            n141 = property class="MCListbox"(reference=w334, "TopLeft"=w333) -> ()  [unwired: 1 in, 2 out]
          }
        }
      }
      frame "UpdateGraph" {
        n142 = Increment(x=w358) -> (x+1=w350:u16)
        n143 = local read "TestDataCurve"() -> (w355:dbl[][])
        n144 = Increment(x=w356) -> (x+1=w352:u16)
        n145 = Increment(x=w357) -> (x+1=w351:u16)
        n146 = Increment(x=w359) -> (x+1=w349:u16)
        n147 = Index Array(array=w355, index (col) #1=w353, index (col) #2=w352, index (col) #3=w351, index (col) #4=w350, index (col) #5=w349) -> (element #1=w365:dbl[], element #2=w366:dbl[], element #3=w367:dbl[], element #4=w368:dbl[], element #5=w369:dbl[])  [unwired: 5 in]
        n148 = Bundle("TestDataCurve"=w365, "TestDataCurve"=w366) -> (w364:T6)  [unwired: 1 in]
        n149 = Bundle("TestDataCurve"=w365, "TestDataCurve"=w367) -> (w363:T6)  [unwired: 1 in]
        n150 = Bundle("TestDataCurve"=w365, "TestDataCurve"=w368) -> (w362:T6)  [unwired: 1 in]
        n151 = Bundle("TestDataCurve"=w365, "TestDataCurve"=w369) -> (w361:T6)  [unwired: 1 in]
        n152 = Build Array(w364, w363, w362, w361) -> (w360:T7)
        n153 = property class="XYGraph"(reference=w354, "Value"=w360) -> ()  [unwired: 1 in, 2 out]
      }
      frame "Clean" {
        n154 = local write "TestDataCurve"(dbl[][] [] ("TestDataCurve")) -> ()
        n155 = local write "DataNumber"(u32 0 ("DataNumber")) -> ()
        n156 = property class="MCListbox"(reference=w376, "ItemNames"=string[][] [] ("Item Names")) -> ()  [unwired: 1 in, 2 out]
        n157 = property class="XYGraph"(reference=w374, "Value"=T3 []) -> ()  [unwired: 1 in, 2 out]
        n158 = local write "TestData1D"(dbl[] [] ("TestDataCurve")) -> ()
      }
      frame "End" {
        n159 = local read "StopPlotDataEvn"() -> (w378:refnum<user-event>)
        n160 = Flush Queue(queue=w383, error in (no error)=w382) -> (queue out=w381:refnum<queue>, error out=w380:errorcluster)  [unwired: 1 out]
        n161 = local read "CleanDataEvn"() -> (w377:refnum<user-event>)
        n162 = Release Queue(queue=w381, error in (no error)=w380) -> ()  [unwired: 1 in, 3 out]
        n163 = Destroy User Event(user event=w378) -> ()  [unwired: 1 in, 1 out]
        n164 = Destroy User Event(user event=w377) -> ()  [unwired: 1 in, 1 out]
      }
    }
  }
  n165 = Unregister For Events(event registration refnum=w14) -> ()  [unwired: 1 in, 1 out]
